vi "rangesStringToArray.vi"(9 "isThere\"-\"?":bool, 11 "String":string) -> (3 "Array":i32[](array[numeric]))   [LabVIEW 2024]
doc: "Converts string (x-y) to array x, x+1, ..., y"
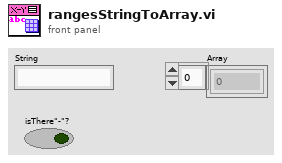
[diagram p1: front panel]
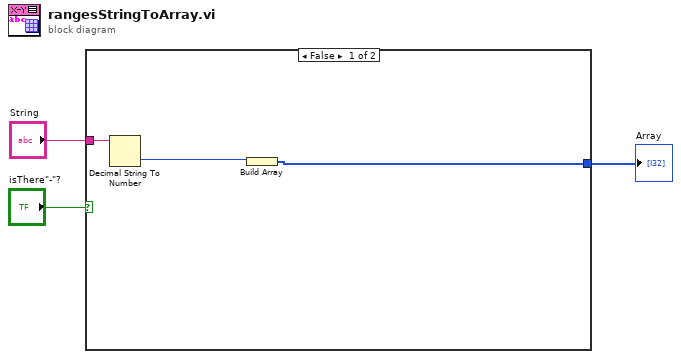
[diagram p0: block diagram]
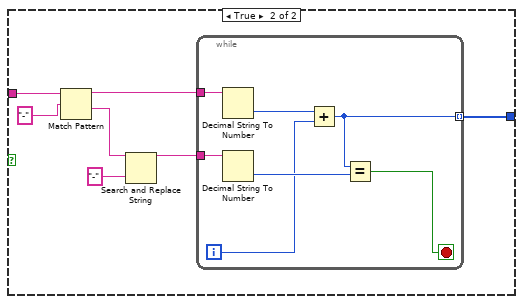
[diagram p2: hidden frame]
diagram:
  n1 = case shown="False" "isThere\"-\"?" {
    tunnel: "String" -> [w6 w13]
    tunnel: [w4 w7] -> w2
    frame False {
      n2 = Decimal String To Number(string=w6) -> (number=w5:i32)  [unwired: 2 in, 1 out]
      n3 = Build Array(w5) -> (w4:i32[])
    }
    frame True {
      n4 = Match Pattern(string=w13, regular expression="-") -> (before substring=w8:string, after substring=w9:string)  [unwired: 1 in, 2 out]
      n5 = Search and Replace String(input string=w9, search string="-") -> (result string=w10:string)  [unwired: 6 in, 3 out]
      n6 = while {
        tunnel: w10 -> [w19]
        tunnel: w8 -> [w20]
        tunnel: [w14] -> w7 mode=indexing
        i -> [w15]
        stop <- w17 stop-if-true
        n7 = Decimal String To Number(string=w20) -> (number=w16:i32)  [unwired: 2 in, 1 out]
        n8 = Decimal String To Number(string=w19) -> (number=w18:i32)  [unwired: 2 in, 1 out]
        n9 = Add(x=w16, y=w15) -> (x+y=w14:i32)
        n10 = Equal?(x=w14, y=w18) -> (x = y?=w17:bool)
      }
    }
  }
  "Array" <- w2
